vi "close_data_log.vi"(8 "error in (no error)":errorcluster, 11 "lfield_logger in":refnum<class "lfield_logger.lvclass">) -> (0 "error out":errorcluster, 3 "lfield_logger out":refnum<class "lfield_logger.lvclass">)   [LabVIEW 2015, in "lfield_logger.lvclass"]
uses:
  lfield_logger.lvclass
  lfield_logger.lvclass/lfield_logger.ctl
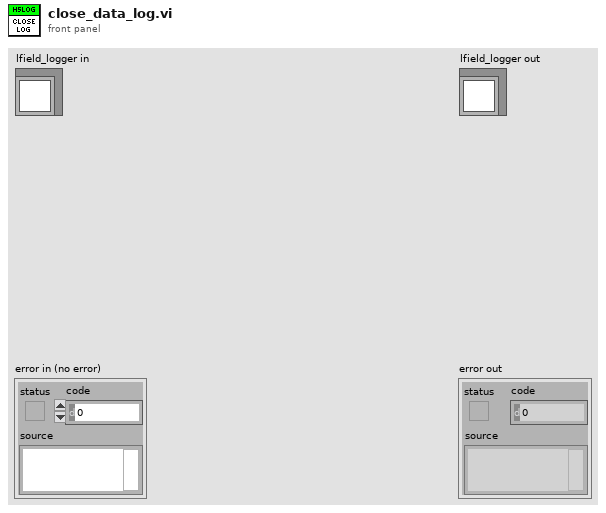
[diagram p1: front panel]
types:
  T1 = typedef "HDF5 Ref.ctl" = refnum<k1>
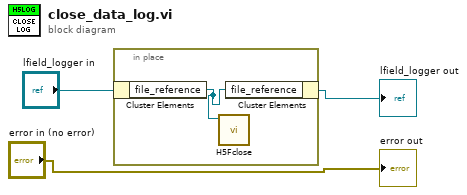
[diagram p0: block diagram]
diagram:
  n1 = in-place {
    n2 = in-place-cluster #1("lfield_logger in") -> ("file_reference"=w4:T1)
    n3 = call <vilib>:"H5Fclose.vi"("HDF5 Ref"=w4) -> ()  [unwired: 8 in, 1 out]
    n4 = in-place-cluster #1("file_reference"=w4) -> (→"lfield_logger out":refnum<class "lfield_logger.lvclass">)
  }
  "error out" <- "error in (no error)"
